vi "AdvServoEventClose.vi"(8 "error in (no error)":errorcluster, 10 "Event Registration Refnum In":refnum<event-registration>, 11 "Device In":i32) -> (0 "error out":errorcluster, 3 "Device Out":i32)   [LabVIEW 2012]
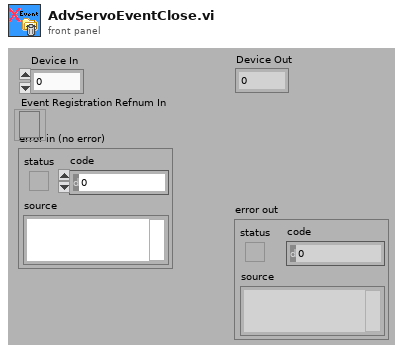
[diagram p1: front panel]
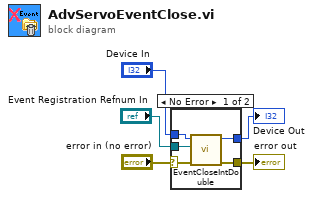
[diagram p0: block diagram]
diagram:
  n1 = case shown="No Error" "error in (no error)" {
    selector: "error in (no error)" -> [w8 w12]
    tunnel: [w7 w12] -> w4
    tunnel: "Device In" -> [w10 w11]
    tunnel: [w9 w11] -> w2
    tunnel: "Event Registration Refnum In" -> [w6 _]
    frame No Error {
      n2 = call "EventCloseIntDouble.vi"("error in (no error)"=w8, "Event Registration Refnum In"=w6, "Device In"=w10) -> ("error out"=w7:errorcluster, "Device Out"=w9:i32)  [unwired: 7 in]
    }
    frame Error {
    }
  }
  "Device Out" <- w2
  "error out" <- w4
